vi "DIO Set.vi"(7 "Box ID":u8, 8 "error in (no error)":errorcluster, 9 "DIO Enable":bool[](array[boolean]), 10 "DIO Direction":bool[](array[boolean]), 11 "BS120x in":refnum<class "BS120x.lvclass">) -> (0 "error out":errorcluster, 3 "BS120x out":refnum<class "BS120x.lvclass">)   [LabVIEW 2021, in "BS120x Driver.lvlib" / "BS120x.lvclass"]
doc: "Sets the direction and status of the DIO on the Battery Simulator 1200.\n(c) 2019 Bloomy Controls, Inc. All rights reserved."
uses:
  BS120x.lvclass
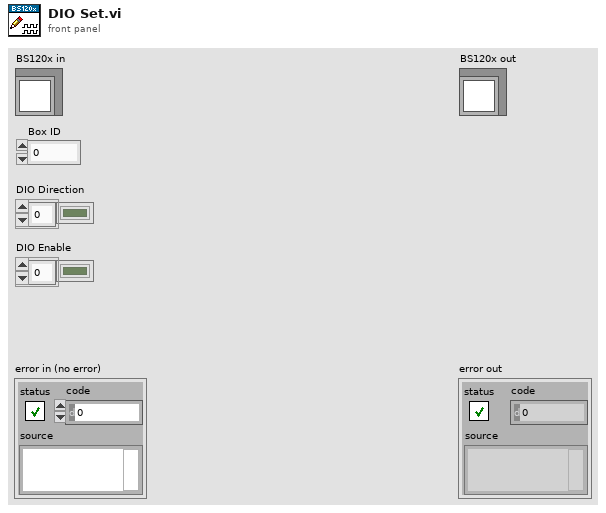
[diagram p1: front panel]
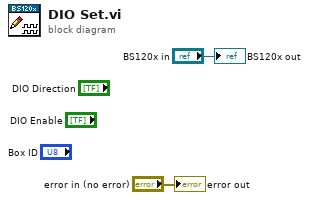
[diagram p0: block diagram]
diagram:
  "error out" <- "error in (no error)"
  "BS120x out" <- "BS120x in"
